vi "List Classes.vi"(8 "Error In":errorcluster, 11 "Application In":refnum<class "Application.lvclass">) -> (0 "Error Out":errorcluster, 2 "List of classes":T1[](array[typedef]), 3 "Application Out":refnum<class "Application.lvclass">)   [LabVIEW 2023, in "Application.lvclass"]
uses:
  Application.lvclass
  Typedef/DVR ref.ctl
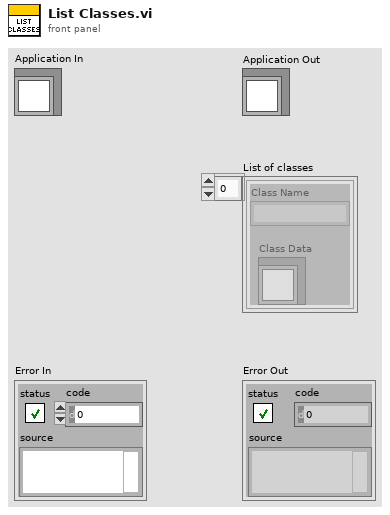
[diagram p1: front panel]
types:
  T1 = typedef "DVR ref.ctl" = cluster{"Class Name":string, "Class Data":refnum<class "Application.lvclass">}
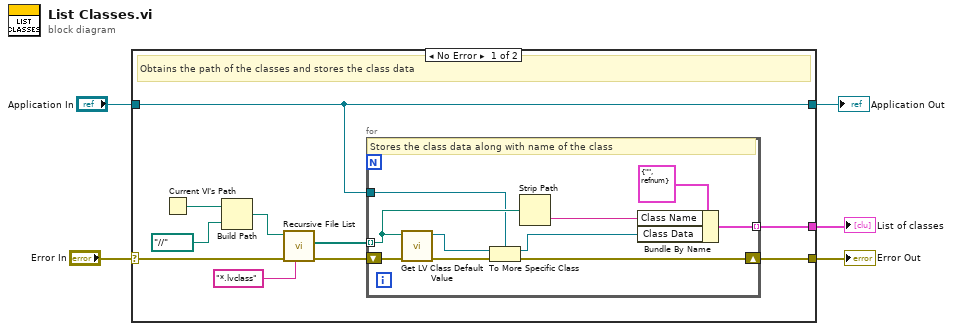
[diagram p0: block diagram]
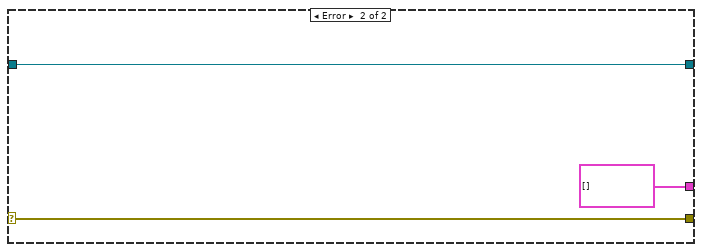
[diagram p2: hidden frame]
diagram:
  n1 = case shown="No Error" "Error In" {
    selector: "Error In" -> [w15 w28]
    tunnel: [w9 w28] -> w4
    tunnel: [w7 T1[] []] -> w3
    tunnel: "Application In" -> [w6 w26]
    tunnel: [w6 w26] -> w1
    frame No Error {
      # "Obtains the path of the classes and stores the class data"
      n2 = Current VI's Path() -> (path=w14:path)
      n3 = Build Path(base path=w14, name or relative path=path "../../..") -> (appended path=w12:path)
      n4 = call <vilib>:"Recursive File List.vi"("pattern"="*.lvclass", "error in (no error)"=w15, "Folder Path"=w12) -> ("error out"=w10:errorcluster, "All Files in Dir"=w8:path[])  [unwired: 4 in, 3 out]
      n5 = for {
        shift-right: [w23] -> w9
        shift-left: w10 -> [w25]
        tunnel: w8 -> [w21] mode=indexing
        tunnel: [w18] -> w7 mode=indexing
        tunnel: w6 -> [w16]
        # "Stores the class data along with name of the class"
        n6 = call <vilib>:"Get LV Class Default Value.vi"("error in (no error)"=w25, "class path"=w21) -> ("error out"=w24:errorcluster, "object"=w22:refnum<class>)  [unwired: 8 in]
        n7 = To More Specific Class(target class=w16, reference=w22, error in=w24) -> (specific class reference=w17:refnum<class "Application.lvclass">, error out=w23:errorcluster)
        n8 = Strip Path(path=w21) -> (name=w19:string)  [unwired: 1 out]
        n9 = Bundle By Name(cluster=T1 {"Class Name"="", "Class Data"=refnum}, "Class Name"=w19, "Class Data"=w17) -> (w18:T1)
      }
    }
    frame Error {
    }
  }
  "Error Out" <- w4
  "List of classes" <- w3
  "Application Out" <- w1
